vi "add to sorted list.vi"(10 "string to insert":string, 11 "sorted list in":T1) -> (3 "sorted list out":T1)   [LabVIEW 2013, in "tag bus.lvlib" / "binary search.lvlib"]
doc: "Inserts a single string into an already sorted list."
uses:
  binary search.lvlib
  sorted list.ctl
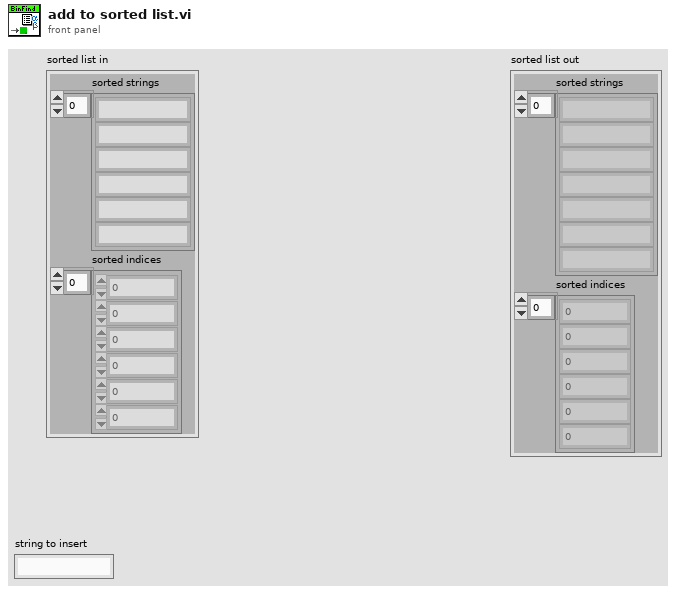
[diagram p1: front panel]
types:
  T1 = typedef "tag bus.lvlib/binary search.lvlib/sorted list.ctl" = cluster{"sorted strings":string[], "sorted indices":i32[]}
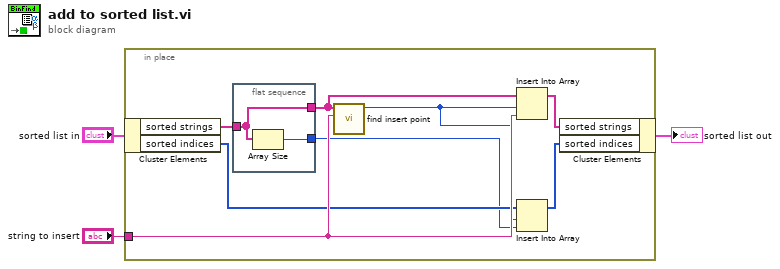
[diagram p0: block diagram]
diagram:
  n1 = in-place {
    in-place-border: "string to insert" -> [w9]
    n2 = in-place-cluster #1("sorted list in") -> ("sorted strings"=w8:string[], "sorted indices"=w6:i32[])
    n3 = flat-sequence {
      tunnel: [w13] -> w5
      tunnel: w8 -> [w12]
      tunnel: [w12] -> w7
      frame #0 {
        n4 = Array Size(array=w12) -> (size(s)=w13:i32)
      }
    }
    n5 = call "find insert point.vi"("string to insert"=w9, "sorted strings"=w7) -> ("index"=w4:i32)  [unwired: 9 in]
    n6 = Insert Into Array(array=w7, index=w4, new element=w9) -> (w11:string[])
    n7 = Insert Into Array(array=w6, index=w4, new element=w5) -> (w10:i32[])
    n8 = in-place-cluster #1("sorted strings"=w11, "sorted indices"=w10) -> (→"sorted list out":T1)
  }
